vi "listCase_v4.vi"() -> ()   [LabVIEW 2019]
doc: "문자열 뒤에서 한 글자 삭제한다.\n한 글자인 경우 0을 출력한다"
panel:
  in  "확인 버튼":bool
  in  "숫자형":dbl
  out "리스트박스":i32(listbox)
  out "문자열":string="0"
  in  "calculator":T1
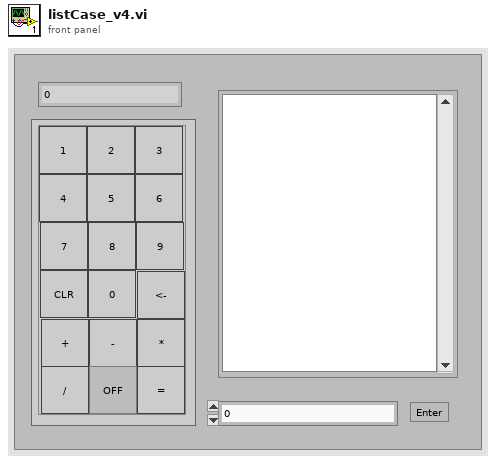
[diagram p1: front panel]
types:
  T1 = cluster{"0":bool, "1":bool, "2":bool, "3":bool, "4":bool, "5":bool, "6":bool, "7":bool, "8":bool, "9":bool, "CLR":bool, "=":bool, "+":bool, "-":bool, "*":bool, "/":bool, "OFF":bool, "<-":bool}
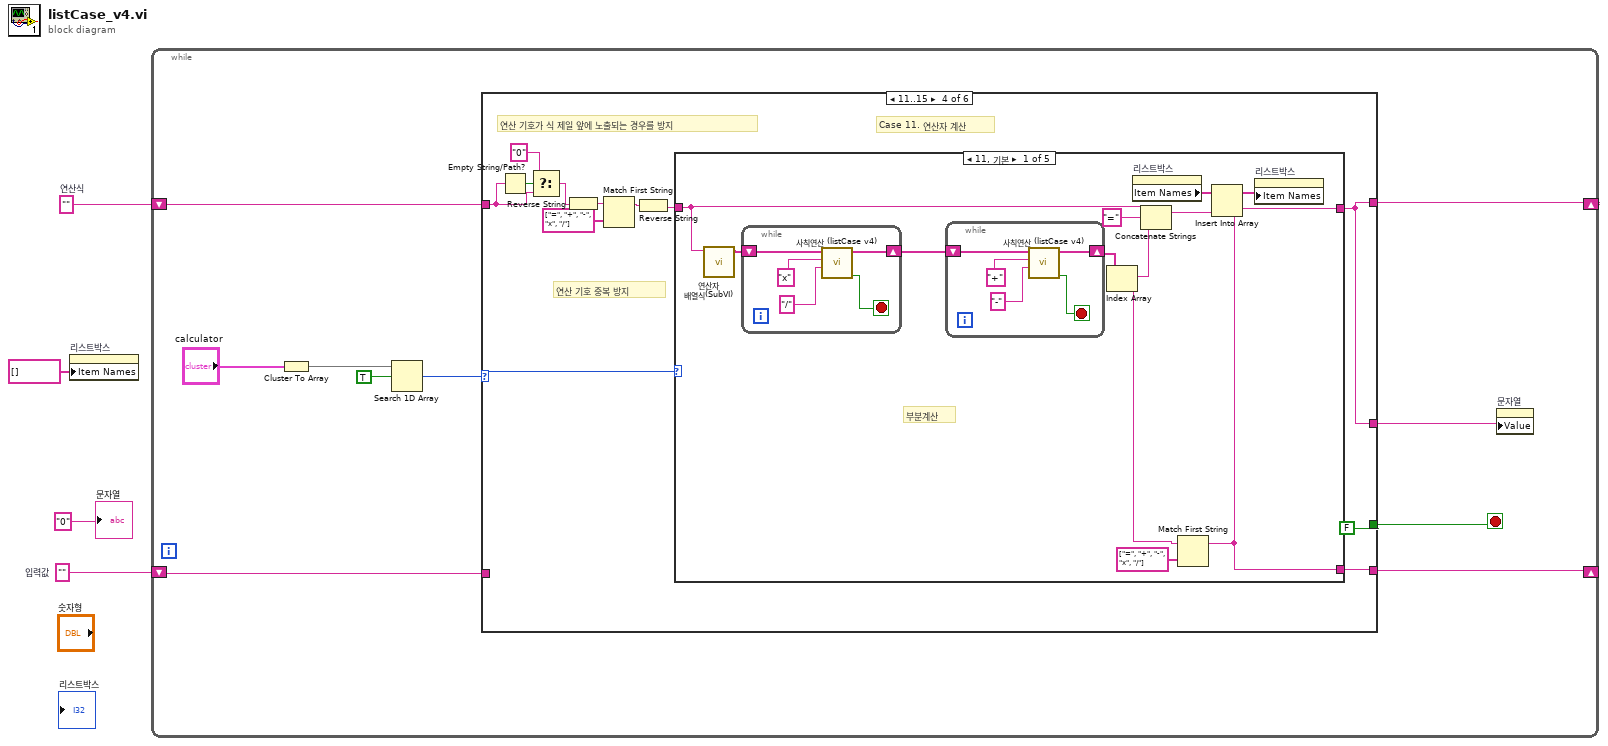
[diagram p0: block diagram]
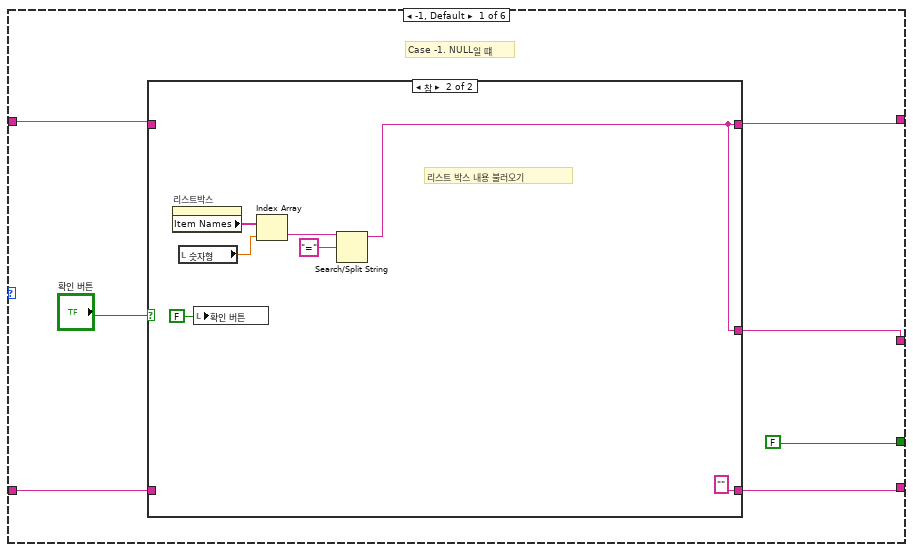
[diagram p2: hidden frame]
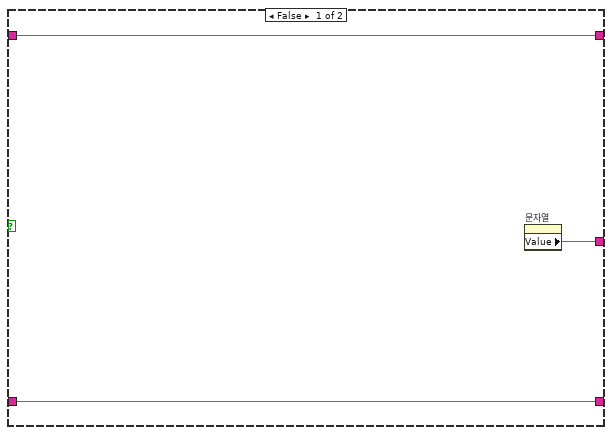
[diagram p3: hidden frame]
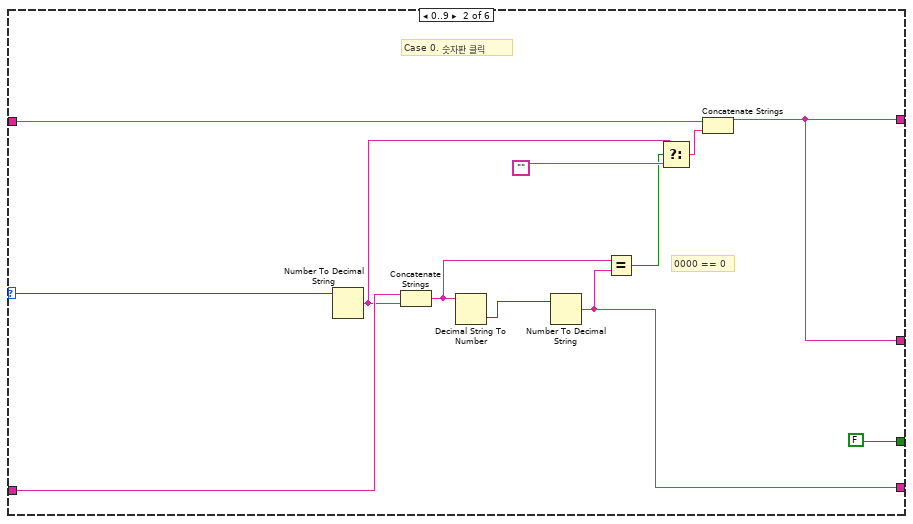
[diagram p4: hidden frame]
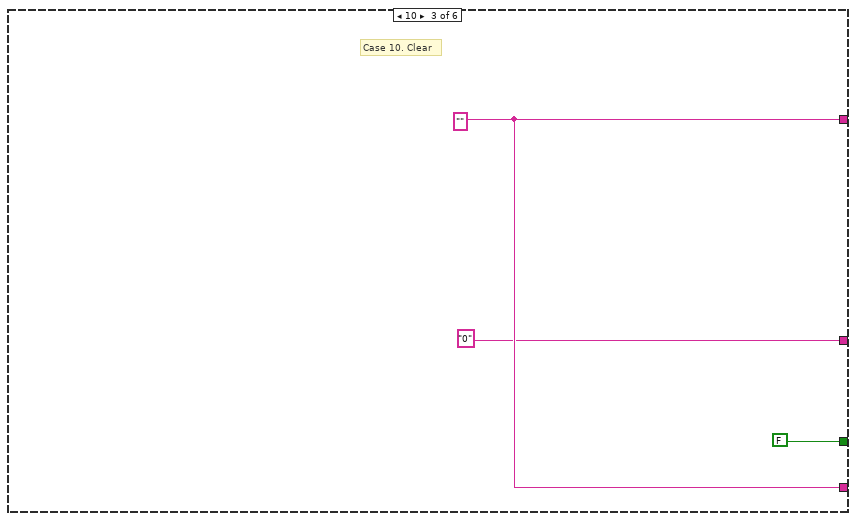
[diagram p5: hidden frame]
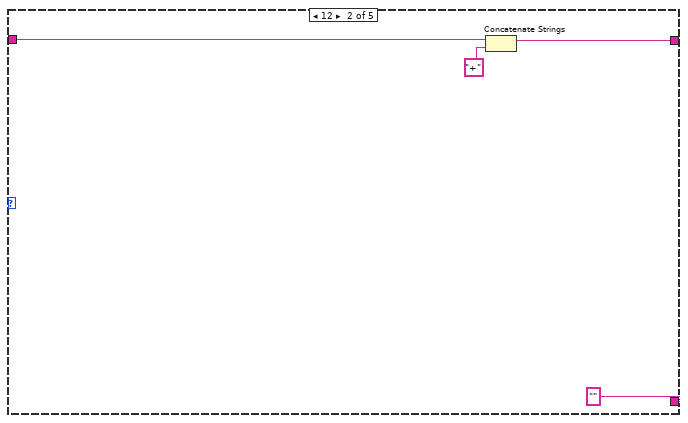
[diagram p6: hidden frame]
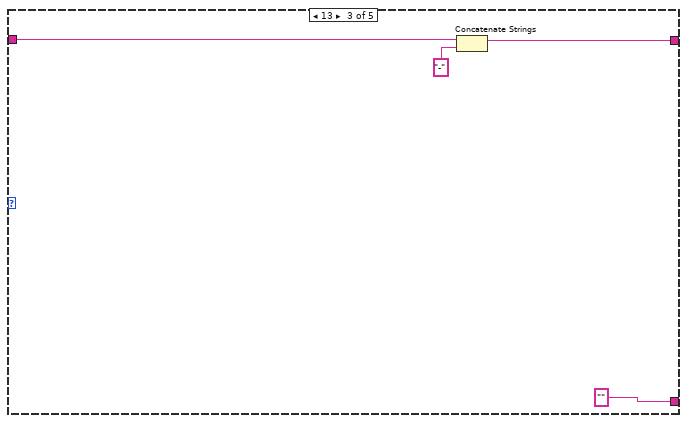
[diagram p7: hidden frame]
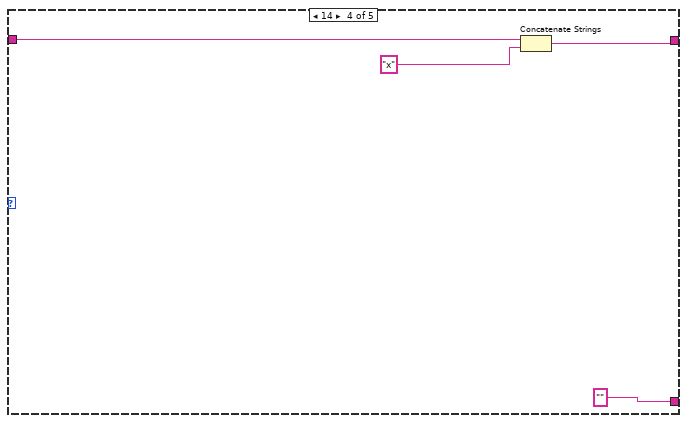
[diagram p8: hidden frame]
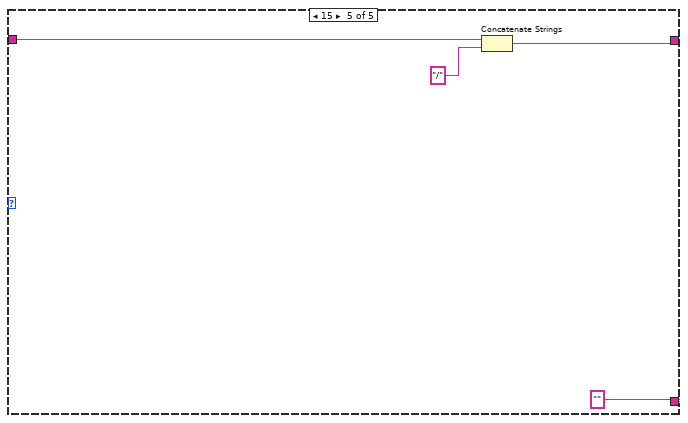
[diagram p9: hidden frame]
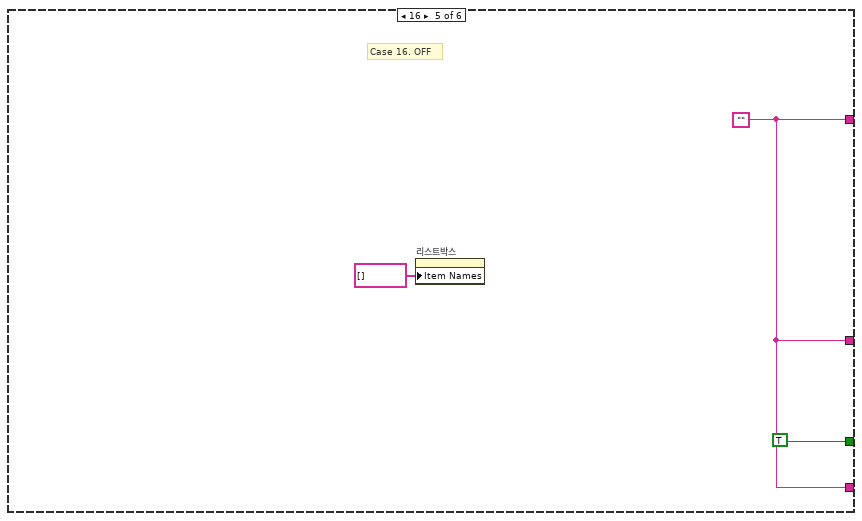
[diagram p10: hidden frame]
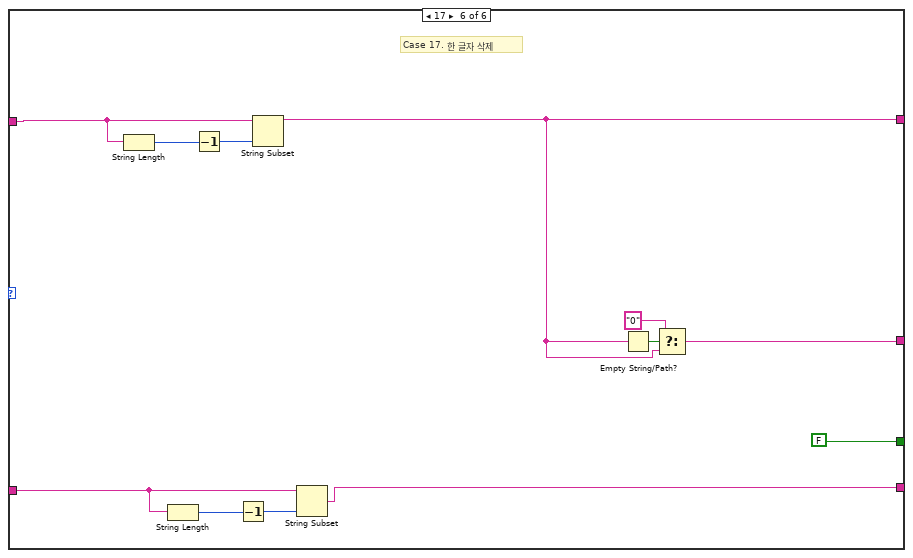
[diagram p11: hidden frame]
diagram:
  w3 = ""  # 연산식
  w4 = ""  # 입력값
  n1 = property on="리스트박스" class="LstBox (엄격한)"("Item Names"=string[] [] ("아이템 이름")) -> ()  [unwired: 2 in, 2 out]
  n2 = while {
    shift-right: [w12] -> _
    shift-left: w4 -> [w13]
    shift-right: [w6] -> _
    shift-left: w3 -> [w7]
    stop <- w9 stop-if-true
    n3 = Cluster To Array(cluster="calculator") -> (array=w10:bool[])
    n4 = Search 1D Array(1D array=w10, element=TRUE ("원소")) -> (index of element=w8:i32)  [unwired: 1 in]
    n5 = case shown="11..15" w8 {
      selector: w8 -> [_ w34 _ w57 _ _]
      tunnel: w13 -> [w21 w43 _ _ _ w106]
      tunnel: [w18 w33 w45 w56 w97 w109] -> w12
      tunnel: [FALSE FALSE FALSE FALSE TRUE FALSE] -> w9
      tunnel: [w17 w35 "0" ("연산식") w55 w97 w99] -> w5
      tunnel: w7 -> [w20 w41 _ w48 _ w103]
      tunnel: [w19 w35 w45 w55 w97 w101] -> w6
      frame -1, Default {
        # "Case -1. NULL일 떄"
        n6 = case shown="참" "확인 버튼" {
          tunnel: w21 -> [w23 _]
          tunnel: w20 -> [w24 _]
          tunnel: [w24 w27] -> w19
          tunnel: [w23 "" ("오프셋(0)")] -> w18
          tunnel: [w22 w27] -> w17
          frame False {
            n7 = property on="문자열" class="Str"() -> ("Value"=w22:string)  [unwired: 2 in, 2 out]
          }
          frame True {
            # "리스트 박스 내용 불러오기"
            n8 = property on="리스트박스" class="LstBox (엄격한)"() -> ("Item Names"=w31:string[])  [unwired: 2 in, 2 out]
            n9 = local read "숫자형"() -> (w25:dbl)
            n10 = local write "확인 버튼"(FALSE) -> ()
            n11 = Index Array(array=w31, index=w25) -> (element=w30:string)
            n12 = Search/Split String(string=w30, search string/char (-)="=" ("검색 문자열/문자 (-)")) -> (substring before match=w27:string)  [unwired: 1 in, 2 out]
          }
        }
      }
      frame 0..9 {
        # "0000 == 0"
        # "Case 0. 숫자판 클릭"
        n13 = Number To Decimal String(number=w34) -> (decimal integer string=w37:string)  [unwired: 1 in]
        n14 = Concatenate Strings(w43, w37) -> (w32:string)
        n15 = Decimal String To Number(string=w32) -> (number=w40:i32)  [unwired: 2 in, 1 out]
        n16 = Number To Decimal String(number=w40) -> (decimal integer string=w33:string)  [unwired: 1 in]
        n17 = Equal?(x=w32, y=w33) -> (x = y?=w36:bool)
        n18 = Select(t=w37, s=w36, f="") -> (s? t:f=w38:string)
        n19 = Concatenate Strings(w41, w38) -> (w35:string)
      }
      frame 10 {
        w45 = ""
        # "Case 10. Clear"
      }
      frame 11..15 {
        # "연산 기호 중복 방지"
        # "연산 기호가 식 제일 앞에 노출되는 경우를 방지"
        # "Case 11. 연산자 계산"
        n20 = Empty String/Path?(string/path=w48) -> (empty?=w50:bool)
        n21 = Select(t="0", s=w50, f=w48) -> (s? t:f=w49:string)
        n22 = Reverse String(1:w49) -> (0:w54:string)
        n23 = Match First String(2:string[] ["=", "+", "-", "x", "/"] ("문자열 배열"), 3:w54) -> (1:w53:string)  [unwired: 1 out]
        n24 = Reverse String(1:w53) -> (0:w51:string)
        n25 = case shown="11, 기본" w57 {
          tunnel: [w59 "" "" "" ""] -> w56
          tunnel: [w59 w82 w86 w90 w94] -> w55
          tunnel: w51 -> [w62 w80 w84 w88 w92]
          frame 11, Default {
            # "부분계산"
            n26 = call "연산자 배열식(SubVI).vi"("연산식"=w62) -> ("부분이 삭제된 배열"=w63:string[])  [unwired: 10 in]
            n27 = while {
              shift-right: [w75] -> w65
              shift-left: w63 -> [w79]
              stop <- w76 stop-if-true
              n28 = call "사칙연산 (listCase v4).vi"("연산자 기호 2"="/" ("원소"), "연산자 기호 1"="x" ("원소"), "연산식 문자열"=w79) -> ("계산 완료"=w76:bool, "부분이 삭제된 배열"=w75:string[])  [unwired: 6 in]
            }
            n29 = while {
              shift-right: [w73] -> w64
              shift-left: w65 -> [w74]
              stop <- w72 stop-if-true
              n30 = call "사칙연산 (listCase v4).vi"("연산자 기호 2"="-" ("원소"), "연산자 기호 1"="+" ("원소"), "연산식 문자열"=w74) -> ("계산 완료"=w72:bool, "부분이 삭제된 배열"=w73:string[])  [unwired: 6 in]
            }
            n31 = Index Array(array=w64) -> (element=w60:string)  [unwired: 1 in]
            n32 = property on="리스트박스" class="LstBox (엄격한)"() -> ("Item Names"=w68:string[])  [unwired: 2 in, 2 out]
            n33 = Concatenate Strings(w62, "=", w60) -> (w66:string)
            n34 = Match First String(2:string[] ["=", "+", "-", "x", "/"] ("문자열 배열"), 3:w60) -> (1:w59:string)  [unwired: 1 out]
            n35 = Insert Into Array(array=w68, new element=w66) -> (w67:string[])  [unwired: 1 in]
            n36 = property on="리스트박스" class="LstBox (엄격한)"("Item Names"=w67) -> ()  [unwired: 2 in, 2 out]
          }
          frame 12 {
            n37 = Concatenate Strings(w80, "+") -> (w82:string)
          }
          frame 13 {
            n38 = Concatenate Strings(w84, "-") -> (w86:string)
          }
          frame 14 {
            n39 = Concatenate Strings(w88, "x") -> (w90:string)
          }
          frame 15 {
            n40 = Concatenate Strings(w92, "/") -> (w94:string)
          }
        }
      }
      frame 16 {
        w97 = ""
        # "Case 16. OFF"
        n41 = property on="리스트박스" class="LstBox (엄격한)"("Item Names"=string[] [] ("아이템 이름")) -> ()  [unwired: 2 in, 2 out]
      }
      frame 17 {
        # "Case 17. 한 글자 삭제"
        n42 = String Length(string=w103) -> (length=w104:i32)
        n43 = String Length(string=w106) -> (length=w108:i32)
        n44 = Decrement(x=w104) -> (x-1=w105:i32)
        n45 = Decrement(x=w108) -> (x-1=w107:i32)
        n46 = String Subset(string=w103, length (rest)=w105) -> (substring=w101:string)  [unwired: 1 in]
        n47 = String Subset(string=w106, length (rest)=w107) -> (substring=w109:string)  [unwired: 1 in]
        n48 = Empty String/Path?(string/path=w101) -> (empty?=w102:bool)
        n49 = Select(t="0", s=w102, f=w101) -> (s? t:f=w99:string)
      }
    }
    n50 = property on="문자열" class="Str"("Value"=w5) -> ()  [unwired: 2 in, 2 out]
  }
  "문자열" <- "0"
